vi "Set channel parameters.vi"(8 "error in (no error)":errorcluster, 11 "Channel Sub in":refnum<class "Channel Sub.lvclass">) -> (0 "error out":errorcluster, 3 "Channel Sub out":refnum<class "Channel Sub.lvclass">)   [LabVIEW 2018, in "Channel Sub.lvclass"]
uses:
  Channel Sub.lvclass
  <vilib>/addons/zeromq/socket_type.ctl
  Communication Channel/Communication Channel.lvclass
  Socket/Socket.lvclass
  <vilib>/addons/zeromq/zeromq.lvlib
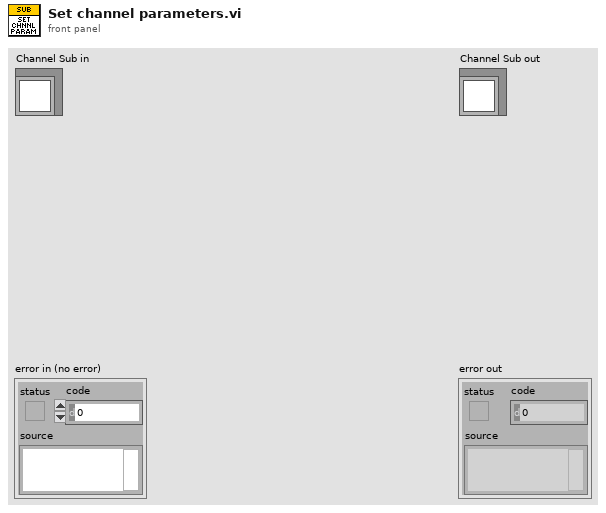
[diagram p1: front panel]
types:
  T1 = typedef "zeromq.lvlib/socket_type.ctl" = enum8{"ZMQ_PAIR", "ZMQ_PUB", "ZMQ_SUB", "ZMQ_REQ", "ZMQ_REP", "ZMQ_DEALER", "ZMQ_ROUTER", "ZMQ_PULL", "ZMQ_PUSH", "ZMQ_XPUB", "ZMQ_XSUB", "ZMQ_STREAM", "ZMQ_SERVER", "ZMQ_CLIENT", "ZMQ_RADIO", "ZMQ_DISH", "ZMQ_GATHER", "ZMQ_SCATTER", "ZMQ_DGRAM"}
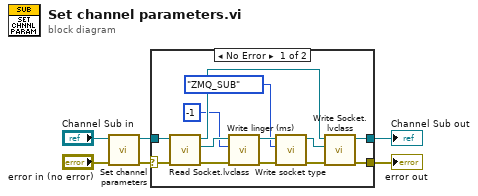
[diagram p0: block diagram]
diagram:
  n1 = call-parent "Set channel parameters.vi"("error in (no error)"="error in (no error)", "Communication Channel in"="Channel Sub in") -> ("error out"=w3:errorcluster, "Communication Channel out"=w4:refnum<class "Channel Sub.lvclass">)  [unwired: 8 in]
  n2 = case shown="No Error" w3 {
    selector: w3 -> [w18 w20]
    tunnel: w4 -> [w19 w21]
    tunnel: [w16 w21] -> w2
    tunnel: [w15 w20] -> w1
    frame No Error {
      n3 = call-dynamic "Read Socket.lvclass.vi"("error in (no error)"=w18, "Communication Channel in"=w19) -> ("error out"=w9:errorcluster, "Socket.lvclass"=w14:refnum<class "Socket.lvclass">, "Communication Channel out"=w17:refnum<class "Channel Sub.lvclass">)  [unwired: 7 in]
      n4 = call-dynamic "Write linger (ms).vi"("error in (no error)"=w9, "linger (ms)"=-1, "Socket in"=w14) -> ("error out"=w10:errorcluster, "Socket out"=w13:refnum<class "Socket.lvclass">)  [unwired: 7 in]
      n5 = call-dynamic "Write socket type.vi"("error in (no error)"=w10, "Socket type"=socket_type."ZMQ_SUB", "Socket in"=w13) -> ("error out"=w11:errorcluster, "Socket out"=w12:refnum<class "Socket.lvclass">)  [unwired: 7 in]
      n6 = call-dynamic "Write Socket.lvclass.vi"("error in (no error)"=w11, "Socket2.lvclass"=w12, "Communication Channel in"=w17) -> ("error out"=w15:errorcluster, "Communication Channel out"=w16:refnum<class "Channel Sub.lvclass">)  [unwired: 7 in]
    }
    frame Error {
    }
  }
  "error out" <- w1
  "Channel Sub out" <- w2
